vi "Automatic inc dec stop my logic.vi"() -> ()   [LabVIEW 2021]
panel:
  in  "x":dbl
  in  "stop":bool
  out "y":dbl
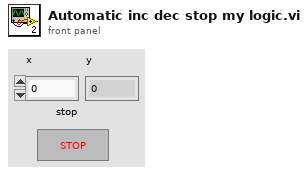
[diagram p1: front panel]
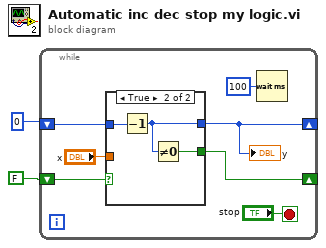
[diagram p0: block diagram]
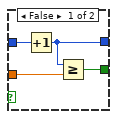
[diagram p2: hidden frame]
diagram:
  n1 = while {
    shift-right: [w8] -> _
    shift-left: FALSE -> [w7]
    shift-right: [w4] -> _
    shift-left: 0 -> [w6]
    stop <- "stop" stop-if-true
    n2 = case shown="True" w7 {
      tunnel: "x" -> [w13 _]
      tunnel: [w12 w15] -> w8
      tunnel: w6 -> [w11 w16]
      tunnel: [w10 w14] -> w4
      frame False {
        n3 = Increment(x=w11) -> (x+1=w10:i32)
        n4 = Greater Or Equal?(x=w10, y=w13) -> (x >= y?=w12:bool)
      }
      frame True {
        n5 = Decrement(x=w16) -> (x-1=w14:i32)
        n6 = Not Equal To 0?(x=w14) -> (x != 0?=w15:bool)
      }
    }
    "y" <- w4
    n7 = Wait (ms)(milliseconds to wait=u32 100 ("millisecond timer value")) -> ()  [unwired: 1 out]
  }
